vi "Read reference.vi"(6 "error in":errorcluster, 9 "GObject in":refnum<class "Generic.lvclass">) -> (0 "error out":errorcluster, 1 "reference":refnum<vi>, 3 "GObject out":refnum<class "Generic.lvclass">)   [LabVIEW 2014, in "Raspberry Pi Compatible Compiler for LabVIEW.lvlib" / "Generic.lvclass"]
uses:
  Generic.lvclass
  Generic.lvclass/Generic.ctl
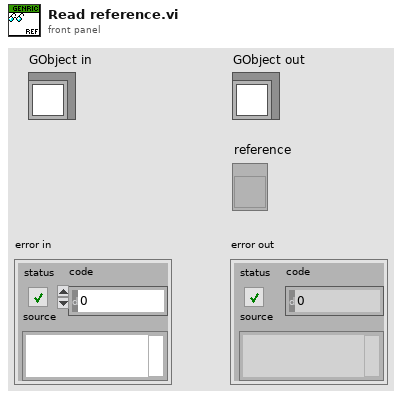
[diagram p1: front panel]
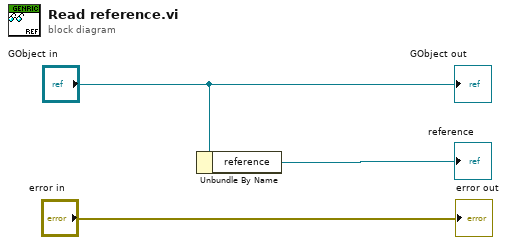
[diagram p0: block diagram]
diagram:
  n1 = Unbundle By Name("GObject in") -> ("reference"=→"reference":refnum<vi>)
  "GObject out" <- "GObject in"
  "error out" <- "error in"
